vi "mlink_ao_scan_init.vi"(4 "data":sgl[](array[numeric]), 5 "mode":enum16{"Periodic", "Stream"}(ring), 6 "channels":u8[](array[numeric]), 7 "range":dbl[](array[numeric]), 8 "error in (no error)":errorcluster, 9 "rate":dbl, 10 "duration":dbl, 11 "connection ID":i32=-1) -> (0 "error out":errorcluster, 3 "connection ID out":i32)   [LabVIEW 2009, in "MicroDAQ.lvlib" / "mlink.lvlib"]
doc: "This function initiates analog output scanning session. The function must be called before \nacquisition is started. The channels argument is an array containing channels numbers \naccording to MicroDAQ hardware configuration. The ch_count argument determines number\nof used channels. The range argument specifies channel output range. An array n-by-2 where\nn is number of used channels shall be provided. In order to obtain supported ranges check your analog output specification. The data argument contains data to be output and is specified as a float array of n x m elements lenght (data_size), where m is the number of scans to generate, and n is the number of used output channels.\nImportant: The data argument determines size of data which can be queued with mlink_ao_scan_data(). Queued data size must be the same size as data argument in mlink_ao_scan_init() function.\nThe rate argument determines scans per second rate for selected analog input channels. \nMinimum value is 1 scan per second, maximum depends on MicroDAQ analog output type. The duration argument specifies a duration of acquisition in seconds. When set to -1, the \nsession will run continuously, writing data until stopped with mlink_ao_scan_stop() function. The stream_mode argument determines scanning session behavior. Two modes are available -periodic and stream.\nThe periodic mode (stream_mode = 0) uses a single buffer which data is output from. When\nthe end of the buffer is reached, data index is switched to the beginning of the buffer. This mode is suitable for generating periodic signals e.g sine waveform. The buffer can be changed during signal generation with mlink_ao_scan_data() function.\nThe stream mode (stream_mode = 1) uses two buffers architecture to ensure uninterrupted analog signal generation. This mode of operation is suitable for stream data type e.g. generating audio stream, this mode requires from user to queue data with certain time \nconstraints. If new data isn't queued on time, last value remains on analog output until new data has been queued."
uses:
  <instrlib>/MicroDAQ/Mlink library wraper/mlink.lvlib
  <instrlib>/MicroDAQ/MLink32.dll
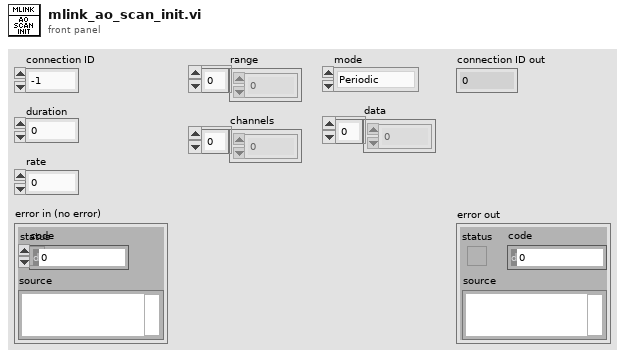
[diagram p1: front panel]
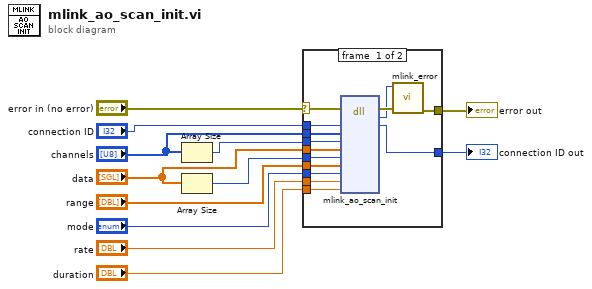
[diagram p0: block diagram]
diagram:
  n1 = Array Size(array="channels") -> (size(s)=w3:i32)
  n2 = Array Size(array="data") -> (size(s)=w6:i32)
  n3 = case shown="No Error" "error in (no error)" {
    selector: "error in (no error)" -> [w24 w28]
    tunnel: "connection ID" -> [w26 w27]
    tunnel: [w25 w27] -> w11
    tunnel: "rate" -> [w23 _]
    tunnel: "duration" -> [w22 _]
    tunnel: "data" -> [w21 _]
    tunnel: w6 -> [w20 _]
    tunnel: "range" -> [w19 _]
    tunnel: [w16 w28] -> w2
    tunnel: "channels" -> [w15 _]
    tunnel: w3 -> [w14 _]
    tunnel: "mode" -> [w13 _]
    frame #0 {
      n4 = dll-call lib="C:/Program Files (x86)/National Instruments/LabVIEW 2009/instr.lib/MicroDAQ/MLink32.dll" fn="mlink_ao_scan_init"(error in=w24, "connection ID"=w26, "channels"=w15, "count"=w14, "data"=w21, "data_size"=w20, "range"=w19, "mode"=w13, "rate"=w23, "duration"=w22) -> (error out=w18:errorcluster, "return type"=w17:i32, "connection ID"=w25:i32)  [unwired: 10 in, 1 out]
      n5 = call <instrlib>:"mlink_error.vi"("error in (no error)"=w18, "error code"=w17) -> ("error out"=w16:errorcluster)  [unwired: 9 in]
    }
    frame #1 {
    }
  }
  "connection ID out" <- w11
  "error out" <- w2
